vi "Last Ack Queue.vi"(10 "Queue":refnum<class "Queue jettl.lvclass">, 11 "Last Ack Queue in":refnum<class "Last Ack Queue.lvclass">) -> (3 "Last Ack Queue out":refnum<class "Last Ack Queue.lvclass">)   [LabVIEW 2021, in "jettl.lvlib" / "jettl Msg Last Ack Queue.lvlib" / "Last Ack Queue.lvclass"]
uses:
  Last Ack Queue.lvclass
  Queue jettl/Queue jettl.lvclass
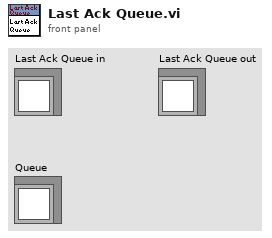
[diagram p1: front panel]
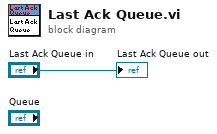
[diagram p0: block diagram]
diagram:
  "Last Ack Queue out" <- "Last Ack Queue in"
